vi "Generate histogram bins.vi"(8 "error in (no error)":errorcluster, 9 "Interval width":sgl, 10 "Maximum value":sgl, 11 "Brigthest bins":i32) -> (0 "error out":errorcluster, 2 "bins array":sgl[](array[numeric]))   [LabVIEW 2012, in "MeritFactor.lvclass"]
uses:
  MeritFactor.lvclass
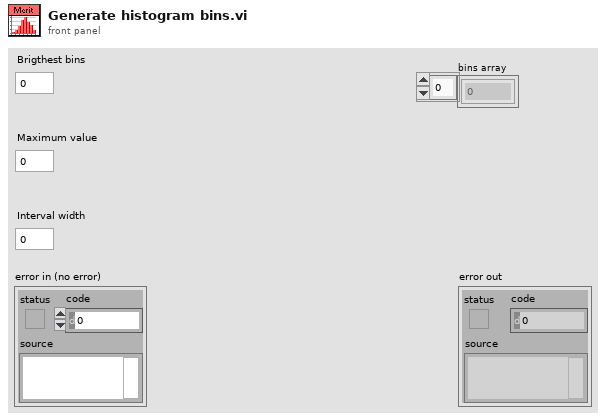
[diagram p1: front panel]
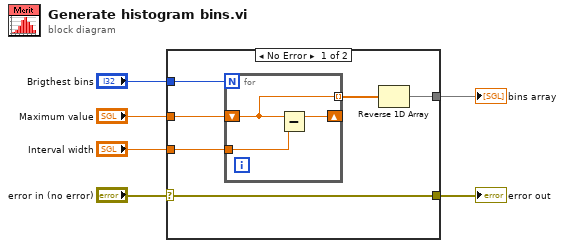
[diagram p0: block diagram]
diagram:
  n1 = case shown="No Error" "error in (no error)" {
    selector: "error in (no error)" -> [w12 w16]
    tunnel: [w12 w16] -> w5
    tunnel: "Brigthest bins" -> [w11 _]
    tunnel: "Maximum value" -> [w10 _]
    tunnel: "Interval width" -> [w9 _]
    tunnel: [w7 _] -> w1
    frame No Error {
      n2 = for {
        N: w11 -> [_]
        shift-right: [w14] -> _
        shift-left: w10 -> [w13]
        tunnel: w9 -> [w15]
        tunnel: [w13] -> w8 mode=indexing
        n3 = Subtract(x=w13, y=w15) -> (x-y=w14:sgl)
      }
      n4 = Reverse 1D Array(array=w8) -> (reversed array=w7:sgl[])
    }
    frame Error {
    }
  }
  "error out" <- w5
  "bins array" <- w1
